vi "MeasAction.vi"(8 "error in (no error)":errorcluster caption="entrée d'erreur (pas d'erreur)", 9 "CurvePointIndex":i32, 10 "AllPointIndex":i32, 11 "InstrClassIn":refnum<class "DAQ6363.lvclass"> caption="DNL_LabVIEW Object in") -> (0 "error out":errorcluster caption="sortie d'erreur", 2 "MeasDatOut":dbl[](array[numeric]), 3 "InstrClassOut":refnum<class "DAQ6363.lvclass"> caption="DNL_LabVIEW Object out")   [LabVIEW 2019, in "DAQ6363.lvclass"]
uses:
  DAQ6363.lvclass
  C:/Programmes Labview/LabScanV1A/DevicesClass/BaseDevice/BaseDevice.lvclass
  DAQ6363.lvclass/DAQ6363.ctl
  <vilib>/DAQmx/read.llb/DAQmx Read (Counter U32 1Chan 1Samp).vi
  <userlib>/GenProg/ReadValByRefBool.vi
  <userlib>/GenProg/ReadValByRefU32.vi
  <vilib>/DAQmx/miscellaneous.llb/DAQmx Fill In Error Info.vi
panel:
  out "ControlsNames":string[](array[string])
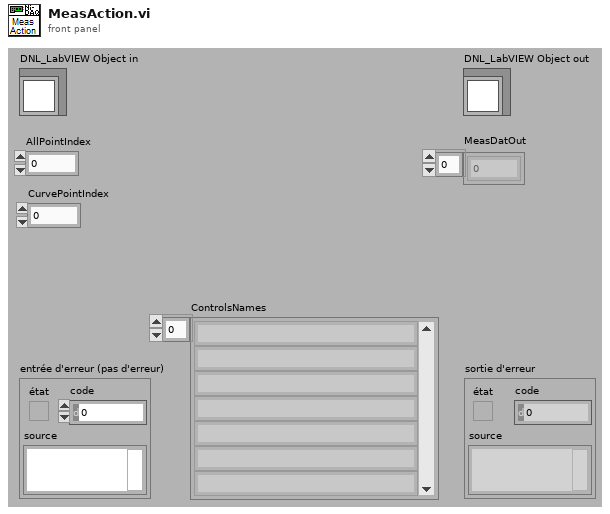
[diagram p1: front panel]
types:
  T1 = typedef "DAQ6363.lvclass/DAQ6363_Func.ctl" = enum16{"CountPulse (Cnt)", "Rabi (Tau) ", "PulsedODMR (Pulses)"}
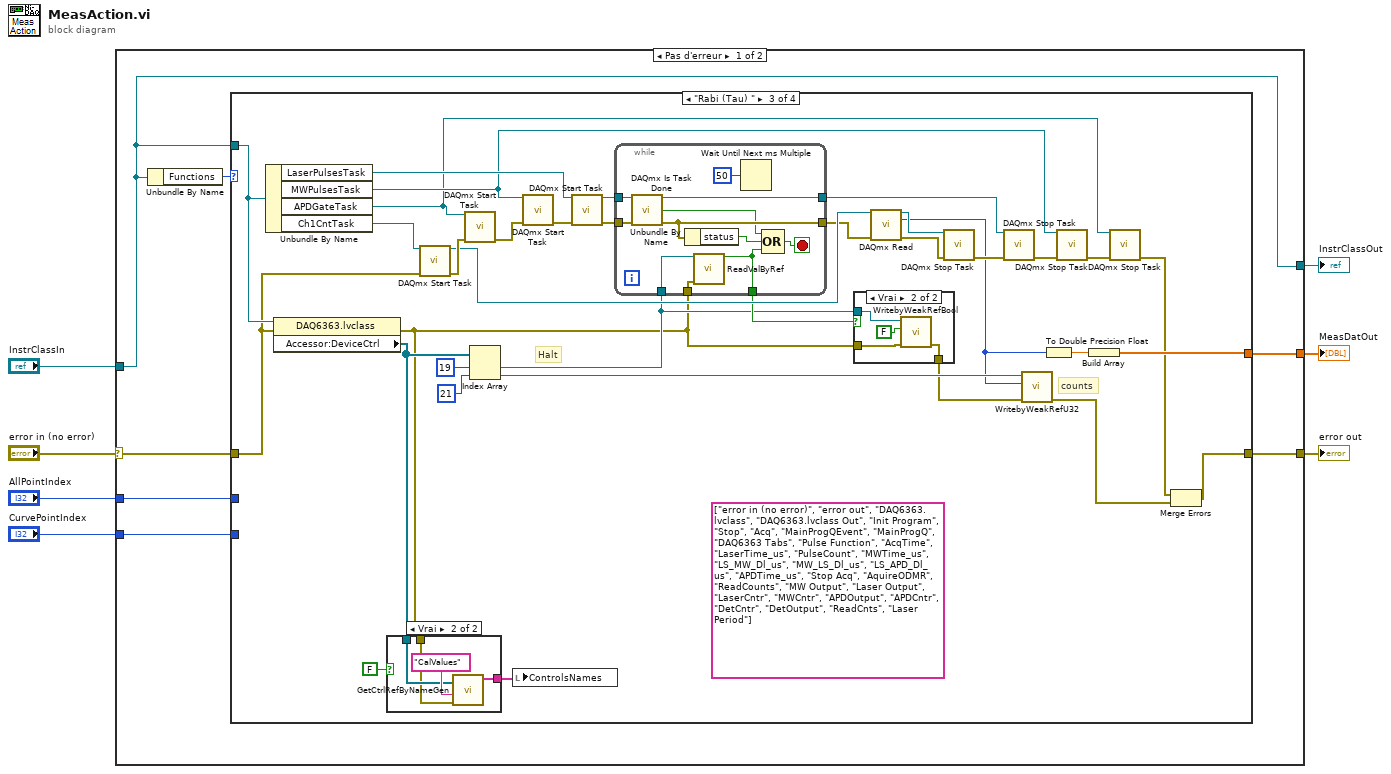
[diagram p0: block diagram]
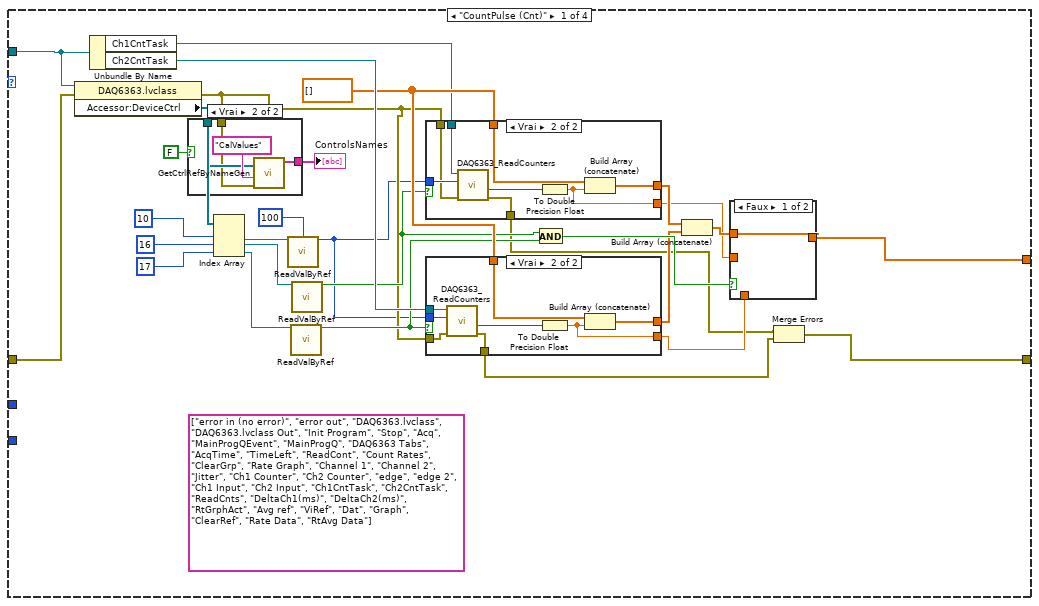
[diagram p2: hidden frame]
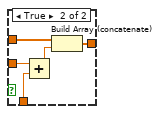
[diagram p4: hidden frame]
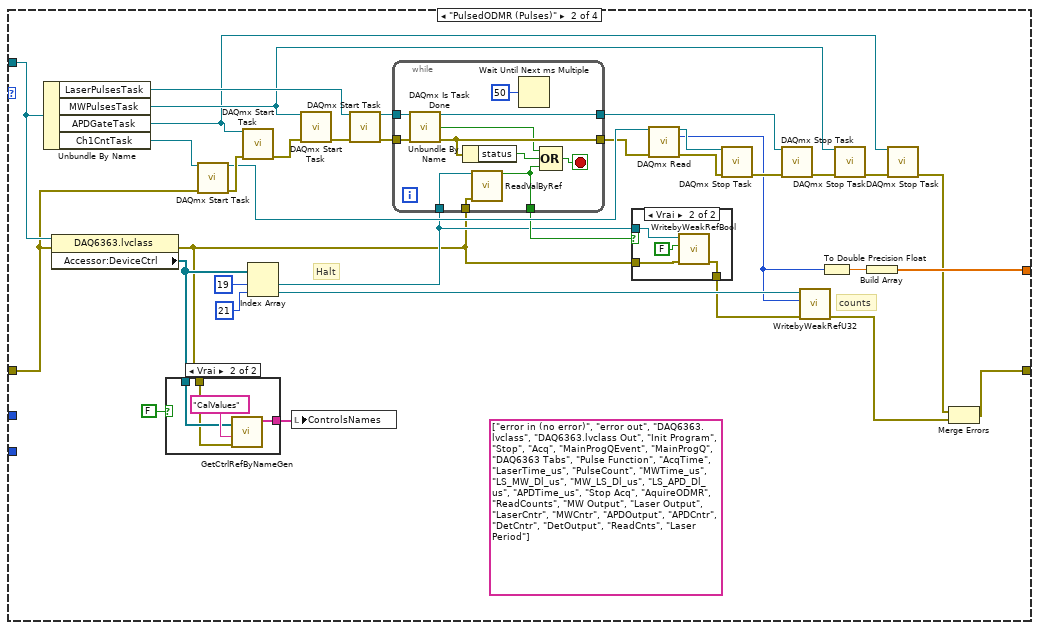
[diagram p7: hidden frame]
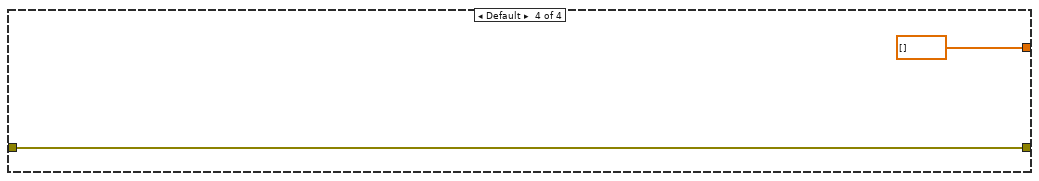
[diagram p12: hidden frame]
diagram:
  n1 = case shown="Pas d'erreur" "error in (no error)" {
    selector: "error in (no error)" -> [w10 w186]
    tunnel: "InstrClassIn" -> [w8 w187]
    tunnel: [w8 w187] -> w5
    tunnel: "AllPointIndex" -> [w14 _]
    tunnel: [w13 w186] -> w3
    tunnel: [w12 _] -> w2
    tunnel: "CurvePointIndex" -> [w9 _]
    frame No Error {
      n2 = Unbundle By Name(w8) -> ("Functions"=w11:T1)
      n3 = case shown="\"Rabi (Tau) \"" w11 {
        tunnel: w14 -> [_ _ _ _]
        tunnel: [w24 w84 w139 w184] -> w13
        tunnel: [w27 w99 w154 dbl[] [] ("Outputs")] -> w12
        tunnel: w10 -> [w41 w87 w142 w184]
        tunnel: w9 -> [_ _ _ _]
        tunnel: w8 -> [w42 w88 w143 _]
        frame "CountPulse (Cnt)" {
          (unwired) string[] ["error in (no error)", "error out", "DAQ6363.lvclass", "DAQ6363.lvclass Out", "Init Program", "Stop", "Acq", "MainProgQEvent", "MainProgQ", "DAQ6363 Tabs", "AcqTime", "TimeLeft", "ReadCont", "Count Rates", "ClearGrp", "Rate Graph", "Channel 1", "Channel 2", "Jitter", "Ch1 Counter", "Ch2 Counter", "edge", "edge 2", "Ch1 Input", "Ch2 Input", "Ch1CntTask", "Ch2CntTask", "ReadCnts", "DeltaCh1(ms)", "DeltaCh2(ms)", "RtGrphAct", "Avg ref", "ViRef", "Dat", "Graph", "ClearRef", "Rate Data", "RtAvg Data"] ("ControlsNames")
          w36 = dbl[] [] ("tableau ajouté")
          n4 = property class="DAQ6363.lvclass"(reference=w42, error in=w41) -> (error out=w20:errorcluster, "Accessor:DeviceCtrl"=w40:refnum<vi>[])  [unwired: 1 out]
          n5 = Unbundle By Name(w42) -> ("Ch1CntTask"=w15:refnum<k21>, "Ch2CntTask"=w37:refnum<k21>)
          n6 = case shown="Vrai" FALSE {
            tunnel: [_ w46] -> w43
            tunnel: w40 -> [_ w45]
            tunnel: w20 -> [_ w44]
            frame False {
            }
            frame True {
              n7 = call <userlib>:"GetCtrlRefByNameGen.vi"("Commandes []"=w45, "ErrorIn(No Error)"=w44, "ControlName"="CalValues") -> ("ControlsNames"=w46:string[])  [unwired: 6 in, 2 out]
            }
          }
          "ControlsNames" <- w43
          n8 = Index Array(array=w40, index #1=10 ("indice"), index #2=16 ("indice"), index #3=17 ("indice")) -> (element #1=w39:refnum<vi>, element #2=w23:refnum<vi>, element #3=w22:refnum<vi>)
          n9 = call-poly <userlib>:"ReadValByRef.vi"("Control Ref"=w39, "Type In"=u32 100 ("Count Period (ms)")) -> ("Valeur"=w19:u32)  [unwired: 12 in, 1 out]
          n10 = call-poly <userlib>:"ReadValByRef.vi"("Control Ref"=w22) -> ("Valeur"=w33:bool)  [unwired: 13 in, 1 out]
          n11 = call-poly <userlib>:"ReadValByRef.vi"("Control Ref"=w23) -> ("Valeur"=w34:bool)  [unwired: 13 in, 1 out]
          n12 = case shown="Vrai" w34 {
            tunnel: w19 -> [_ w73]
            tunnel: [w65 w71] -> w31
            tunnel: w36 -> [w65 w70]
            tunnel: [_ w69] -> w29
            tunnel: [w64 w68] -> w26
            tunnel: w20 -> [w64 w67]
            tunnel: w15 -> [_ w66]
            frame False {
            }
            frame True {
              n13 = call <userlib>:"DAQ6363_ReadCounters.vi"("ErrIn(No Err)"=w67, "Count Period (ms)"=w73, "CntTask"=w66) -> ("ErrOut"=w68:errorcluster, "Counts"=w72:u32)  [unwired: 3 in, 4 out]
              n14 = To Double Precision Float(number=w72) -> (double precision float=w69:dbl)
              n15 = Build Array (concatenate)(w70, w69) -> (w71:dbl[])
            }
          }
          n16 = case shown="Vrai" w33 {
            tunnel: w37 -> [_ w63]
            tunnel: w19 -> [_ w62]
            tunnel: [w55 w60] -> w30
            tunnel: w36 -> [w55 w59]
            tunnel: [_ w58] -> w28
            tunnel: [w54 w57] -> w25
            tunnel: w20 -> [w54 w56]
            frame False {
            }
            frame True {
              n17 = call <userlib>:"DAQ6363_ReadCounters.vi"("ErrIn(No Err)"=w56, "Count Period (ms)"=w62, "CntTask"=w63) -> ("ErrOut"=w57:errorcluster, "Counts"=w61:u32)  [unwired: 3 in, 4 out]
              n18 = To Double Precision Float(number=w61) -> (double precision float=w58:dbl)
              n19 = Build Array (concatenate)(w59, w58) -> (w60:dbl[])
            }
          }
          n20 = And(x=w34, y=w33) -> (x .and. y?=w32:bool)
          n21 = Build Array (concatenate)(w31, w30) -> (w35:dbl[])
          n22 = case shown="Faux" w32 {
            tunnel: w29 -> [_ w53]
            tunnel: w28 -> [_ w52]
            tunnel: w35 -> [w48 w50]
            tunnel: [w48 w49] -> w27
            frame False {
            }
            frame True {
              n23 = Add(x=w53, y=w52) -> (x+y=w51:dbl)
              n24 = Build Array (concatenate)(w50, w51) -> (w49:dbl[])
            }
          }
          n25 = Merge Errors(w26, w25) -> (w24:errorcluster)
        }
        frame "PulsedODMR (Pulses)" {
          (unwired) string[] ["error in (no error)", "error out", "DAQ6363.lvclass", "DAQ6363.lvclass Out", "Init Program", "Stop", "Acq", "MainProgQEvent", "MainProgQ", "DAQ6363 Tabs", "Pulse Function", "AcqTime", "LaserTime_us", "PulseCount", "MWTime_us", "LS_MW_Dl_us", "MW_LS_Dl_us", "LS_APD_Dl_us", "APDTime_us", "Stop Acq", "AquireODMR", "ReadCounts", "MW Output", "Laser Output", "LaserCntr", "MWCntr", "APDOutput", "APDCntr", "DetCntr", "DetOutput", "ReadCnts", "Laser Period"] ("ControlsNames")
          # "Halt"
          # "counts"
          n26 = Unbundle By Name(w88) -> ("LaserPulsesTask"=w108:refnum<k21>, "MWPulsesTask"=w92:refnum<k21>, "APDGateTask"=w90:refnum<k21>, "Ch1CntTask"=w107:refnum<k21>)
          n27 = property class="DAQ6363.lvclass"(reference=w88, error in=w87) -> (error out=w77:errorcluster, "Accessor:DeviceCtrl"=w78:refnum<vi>[])  [unwired: 1 out]
          n28 = case shown="Vrai" FALSE {
            tunnel: [_ w111] -> w76
            tunnel: w78 -> [_ w110]
            tunnel: w77 -> [_ w109]
            frame False {
            }
            frame True {
              n29 = call <userlib>:"GetCtrlRefByNameGen.vi"("Commandes []"=w110, "ErrorIn(No Error)"=w109, "ControlName"="CalValues") -> ("ControlsNames"=w111:string[])  [unwired: 6 in, 2 out]
            }
          }
          n30 = call <vilib>:"DAQmx Start Task.vi"("task/channels in"=w107, "error in"=w87) -> ("task out"=w101:refnum<k21>, "error out"=w103:errorcluster)  [unwired: 12 in]
          n31 = call <vilib>:"DAQmx Start Task.vi"("task/channels in"=w90, "error in"=w103) -> ("error out"=w104:errorcluster)  [unwired: 12 in, 1 out]
          n32 = Index Array(array=w78, index #1=19 ("indice"), index #2=21 ("indice")) -> (element #1=w81:refnum<vi>, element #2=w86:refnum<vi>)
          n33 = local write "ControlsNames"(w76) -> ()
          n34 = call <vilib>:"DAQmx Start Task.vi"("task/channels in"=w92, "error in"=w104) -> ("error out"=w105:errorcluster)  [unwired: 12 in, 1 out]
          n35 = call <vilib>:"DAQmx Start Task.vi"("task/channels in"=w108, "error in"=w105) -> ("task out"=w106:refnum<k21>, "error out"=w102:errorcluster)  [unwired: 12 in]
          n36 = while {
            tunnel: w106 -> [w128]
            tunnel: w102 -> [w127]
            tunnel: [w124] -> w100
            tunnel: [w125] -> w95
            tunnel: w81 -> [w120]
            tunnel: w77 -> [w119]
            tunnel: [w118] -> w82
            stop <- w126 stop-if-true
            n37 = call <vilib>:"DAQmx Is Task Done.vi"("task/channels in"=w128, "error in"=w127) -> ("task out"=w125:refnum<k21>, "task done?"=w121:bool, "error out"=w124:errorcluster)  [unwired: 11 in]
            n38 = Unbundle By Name(w124) -> ("status"=w123:bool)
            n39 = call-poly <userlib>:"ReadValByRef.vi"("Control Ref"=w120, "error in"=w119) -> ("Valeur"=w118:bool)  [unwired: 12 in, 1 out]
            n40 = Wait Until Next ms Multiple(millisecond multiple=u32 50 ("n millisecondes")) -> ()  [unwired: 1 out]
            n41 = Compound Arithmetic op=OR(w121, w123, w118) -> (w126:bool)
          }
          n42 = case shown="Vrai" w82 {
            tunnel: w81 -> [_ w117]
            tunnel: [w113 w115] -> w80
            tunnel: w77 -> [w113 w114]
            frame False {
            }
            frame True {
              n43 = call <userlib>:"WritebyWeakRefBool.vi"("error in"=w114, "Valeur"=FALSE, "Control Ref"=w117) -> ("error out"=w115:errorcluster)  [unwired: 8 in]
            }
          }
          n44 = call-poly <vilib>:"DAQmx Read.vi"("task/channels in"=w101, "error in"=w100) -> ("task out"=w96:refnum<k21>, "data"=w85:u32, "error out"=w97:errorcluster)  [unwired: 11 in]
          n45 = call <vilib>:"DAQmx Stop Task.vi"("task/channels in"=w96, "error in"=w97) -> ("error out"=w94:errorcluster)  [unwired: 12 in, 1 out]
          n46 = call <vilib>:"DAQmx Stop Task.vi"("task/channels in"=w95, "error in"=w94) -> ("error out"=w93:errorcluster)  [unwired: 12 in, 1 out]
          n47 = call <userlib>:"WritebyWeakRefU32.vi"("error in"=w80, "Valeur"=w85, "Control Ref"=w86) -> ("error out"=w83:errorcluster)  [unwired: 8 in]
          n48 = To Double Precision Float(number=w85) -> (double precision float=w98:dbl)
          n49 = call <vilib>:"DAQmx Stop Task.vi"("task/channels in"=w92, "error in"=w93) -> ("error out"=w91:errorcluster)  [unwired: 12 in, 1 out]
          n50 = Build Array(w98) -> (w99:dbl[])
          n51 = call <vilib>:"DAQmx Stop Task.vi"("task/channels in"=w90, "error in"=w91) -> ("error out"=w89:errorcluster)  [unwired: 12 in, 1 out]
          n52 = Merge Errors(w89, w83) -> (w84:errorcluster)
        }
        frame "Rabi (Tau) " {
          (unwired) string[] ["error in (no error)", "error out", "DAQ6363.lvclass", "DAQ6363.lvclass Out", "Init Program", "Stop", "Acq", "MainProgQEvent", "MainProgQ", "DAQ6363 Tabs", "Pulse Function", "AcqTime", "LaserTime_us", "PulseCount", "MWTime_us", "LS_MW_Dl_us", "MW_LS_Dl_us", "LS_APD_Dl_us", "APDTime_us", "Stop Acq", "AquireODMR", "ReadCounts", "MW Output", "Laser Output", "LaserCntr", "MWCntr", "APDOutput", "APDCntr", "DetCntr", "DetOutput", "ReadCnts", "Laser Period"] ("ControlsNames")
          # "Halt"
          # "counts"
          n53 = Unbundle By Name(w143) -> ("LaserPulsesTask"=w163:refnum<k21>, "MWPulsesTask"=w147:refnum<k21>, "APDGateTask"=w145:refnum<k21>, "Ch1CntTask"=w162:refnum<k21>)
          n54 = property class="DAQ6363.lvclass"(reference=w143, error in=w142) -> (error out=w132:errorcluster, "Accessor:DeviceCtrl"=w133:refnum<vi>[])  [unwired: 1 out]
          n55 = case shown="Vrai" FALSE {
            tunnel: [_ w166] -> w131
            tunnel: w133 -> [_ w165]
            tunnel: w132 -> [_ w164]
            frame False {
            }
            frame True {
              n56 = call <userlib>:"GetCtrlRefByNameGen.vi"("Commandes []"=w165, "ErrorIn(No Error)"=w164, "ControlName"="CalValues") -> ("ControlsNames"=w166:string[])  [unwired: 6 in, 2 out]
            }
          }
          n57 = call <vilib>:"DAQmx Start Task.vi"("task/channels in"=w162, "error in"=w142) -> ("task out"=w156:refnum<k21>, "error out"=w158:errorcluster)  [unwired: 12 in]
          n58 = call <vilib>:"DAQmx Start Task.vi"("task/channels in"=w145, "error in"=w158) -> ("error out"=w159:errorcluster)  [unwired: 12 in, 1 out]
          n59 = Index Array(array=w133, index #1=19 ("indice"), index #2=21 ("indice")) -> (element #1=w136:refnum<vi>, element #2=w141:refnum<vi>)
          n60 = local write "ControlsNames"(w131) -> ()
          n61 = call <vilib>:"DAQmx Start Task.vi"("task/channels in"=w147, "error in"=w159) -> ("error out"=w160:errorcluster)  [unwired: 12 in, 1 out]
          n62 = call <vilib>:"DAQmx Start Task.vi"("task/channels in"=w163, "error in"=w160) -> ("task out"=w161:refnum<k21>, "error out"=w157:errorcluster)  [unwired: 12 in]
          n63 = while {
            tunnel: w161 -> [w183]
            tunnel: w157 -> [w182]
            tunnel: [w179] -> w155
            tunnel: [w180] -> w150
            tunnel: w136 -> [w175]
            tunnel: w132 -> [w174]
            tunnel: [w173] -> w137
            stop <- w181 stop-if-true
            n64 = call <vilib>:"DAQmx Is Task Done.vi"("task/channels in"=w183, "error in"=w182) -> ("task out"=w180:refnum<k21>, "task done?"=w176:bool, "error out"=w179:errorcluster)  [unwired: 11 in]
            n65 = Unbundle By Name(w179) -> ("status"=w178:bool)
            n66 = call-poly <userlib>:"ReadValByRef.vi"("Control Ref"=w175, "error in"=w174) -> ("Valeur"=w173:bool)  [unwired: 12 in, 1 out]
            n67 = Wait Until Next ms Multiple(millisecond multiple=u32 50 ("n millisecondes")) -> ()  [unwired: 1 out]
            n68 = Compound Arithmetic op=OR(w176, w178, w173) -> (w181:bool)
          }
          n69 = case shown="Vrai" w137 {
            tunnel: w136 -> [_ w172]
            tunnel: [w168 w170] -> w135
            tunnel: w132 -> [w168 w169]
            frame False {
            }
            frame True {
              n70 = call <userlib>:"WritebyWeakRefBool.vi"("error in"=w169, "Valeur"=FALSE, "Control Ref"=w172) -> ("error out"=w170:errorcluster)  [unwired: 8 in]
            }
          }
          n71 = call-poly <vilib>:"DAQmx Read.vi"("task/channels in"=w156, "error in"=w155) -> ("task out"=w151:refnum<k21>, "data"=w140:u32, "error out"=w152:errorcluster)  [unwired: 11 in]
          n72 = call <vilib>:"DAQmx Stop Task.vi"("task/channels in"=w151, "error in"=w152) -> ("error out"=w149:errorcluster)  [unwired: 12 in, 1 out]
          n73 = call <vilib>:"DAQmx Stop Task.vi"("task/channels in"=w150, "error in"=w149) -> ("error out"=w148:errorcluster)  [unwired: 12 in, 1 out]
          n74 = call <userlib>:"WritebyWeakRefU32.vi"("error in"=w135, "Valeur"=w140, "Control Ref"=w141) -> ("error out"=w138:errorcluster)  [unwired: 8 in]
          n75 = To Double Precision Float(number=w140) -> (double precision float=w153:dbl)
          n76 = call <vilib>:"DAQmx Stop Task.vi"("task/channels in"=w147, "error in"=w148) -> ("error out"=w146:errorcluster)  [unwired: 12 in, 1 out]
          n77 = Build Array(w153) -> (w154:dbl[])
          n78 = call <vilib>:"DAQmx Stop Task.vi"("task/channels in"=w145, "error in"=w146) -> ("error out"=w144:errorcluster)  [unwired: 12 in, 1 out]
          n79 = Merge Errors(w144, w138) -> (w139:errorcluster)
        }
        frame Default {
        }
      }
    }
    frame Error {
    }
  }
  "error out" <- w3
  "InstrClassOut" <- w5
  "MeasDatOut" <- w2
